vi "main_kill_ugshell.vi"   [LabVIEW 2019]
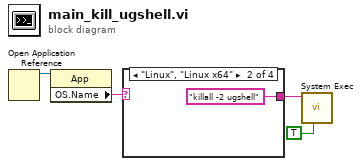
[diagram p0: block diagram]
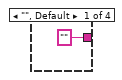
[diagram p2: hidden frame]
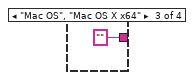
[diagram p3: hidden frame]
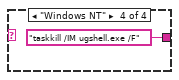
[diagram p4: hidden frame]
diagram:
  n1 = Open Application Reference() -> (3:w4:refnum<vi>)  [unwired: 4 in, 1 out]
  n2 = property class="App"(reference=w4) -> ("OS.Name"=w3:string)  [unwired: 1 in, 2 out]
  n3 = case shown="\"Linux\", \"Linux x64\"" w3 {
    tunnel: ["" ("return type") "killall -2 ugshell" ("command line") "" ("return type") "taskkill /IM ugshell.exe /F" ("command line")] -> w2
    frame "", Default {
    }
    frame "Linux", "Linux x64" {
    }
    frame "Mac OS", "Mac OS X x64" {
    }
    frame "Windows NT" {
    }
  }
  n4 = call <vilib>:"System Exec.vi"("run minimized? (F)"=TRUE, "command line"=w2) -> ()  [unwired: 6 in, 4 out]
